vi "Test DataGrid.vi"() -> ()   [LabVIEW 2018]
panel:
  in  "Multicolumn Listbox":i32(listbox)
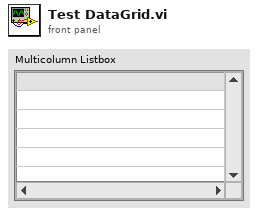
[diagram p1: front panel]
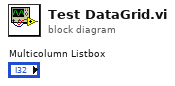
[diagram p0: block diagram]
diagram:
